vi "SystemToggleEnumShift (1).vi"(8 "Enum in":T1, 10 "On/Off":bool, 11 "Stage Complete":bool) -> (0 "Enum":T1)   [LabVIEW 2017]
doc: "Depending on whether subsystems are being activated or deactivated, gives direction to the state machine."
uses:
  SystemToggleEnum.ctl
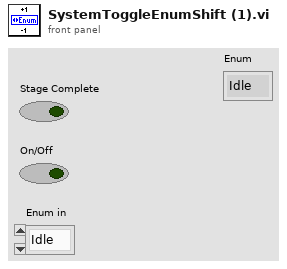
[diagram p1: front panel]
types:
  T1 = typedef "SystemToggleEnum.ctl" = enum16{"Idle", "MagBrake", "Suspension", "Levitation", "Run"}
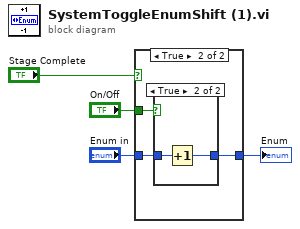
[diagram p0: block diagram]
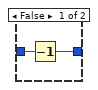
[diagram p3: hidden frame]
diagram:
  n1 = case shown="True" "Stage Complete" {
    tunnel: "Enum in" -> [w5 w7]
    tunnel: "On/Off" -> [_ w8]
    tunnel: [w5 w6] -> w1
    frame False {
    }
    frame True {
      n2 = case shown="True" w8 {
        tunnel: w7 -> [w10 w12]
        tunnel: [w9 w11] -> w6
        frame False {
          n3 = Decrement(x=w10) -> (x-1=w9:T1)
        }
        frame True {
          n4 = Increment(x=w12) -> (x+1=w11:T1)
        }
      }
    }
  }
  "Enum" <- w1
